vi "TFTLCD显示实验.vi"() -> ()   [LabVIEW 2011]
uses:
  <vilib>/STM32_DriverVI_Interface_F4/LCD/Brush Color_Index_F4.ctl
  <vilib>/STM32_DriverVI_Interface_F4/LCD/Font_Size_F4.ctl
  <vilib>/STM32_DriverVI_Interface_F4/LCD/Show_Mode_F4.ctl
  <vilib>/STM32_DriverVI_Interface_F4/LCD/Direction_F4.ctl
  <vilib>/STM32_DriverVI_Interface_F4/LCD/Backlight_F4.ctl
  <vilib>/STM32_DriverVI_Interface_F4/LCD/LCD_Init_F4.vi
panel:
  in  "Display Direction":T1
  in  "停止":bool
  in  "轨迹颜色":T2=enum."Red"
  in  "矩形填充颜色":T2=enum."Magenta（品红）"
  in  "Show_Mode":T3
  in  "Font_Size":T4=enum."Big_Font（16）"
  in  "字体颜色":T2=enum."Magenta（品红）"
  in  "清屏背景色":T2
  in  "String":string="dlw30@126.com"
  in  "Len":u16 max=320
  in  "U32 Number":u32=999999
  out "LCD_ID":u16 format="%x"
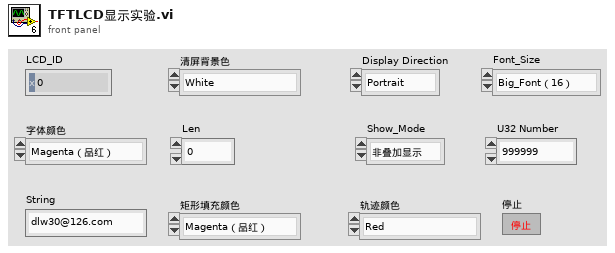
[diagram p1: front panel]
types:
  T1 = typedef "Direction_F4.ctl" = enum8{"Portrait", "Landscape"}
  T2 = typedef "Brush Color_Index_F4.ctl" = enum8{"White", "Black", "Blue", "Green_Blue", "Red", "Magenta（品红）", "Green", "Cyan（青色）", "Yellow", "Brown", "Brown_Red", "Gray", "Dark_Blue", "Light_Blue", "Gray_Blue", "Light_Green", "Light_Gray", "Light_Gray_Blue", "Light_Brown_Blue"}
  T3 = typedef "Show_Mode_F4.ctl" = enum8{"非叠加显示", "叠加显示"}
  T4 = typedef "Font_Size_F4.ctl" = enum8{"Small_Font（12）", "Big_Font（16）"}
  T5 = typedef "Backlight_F4.ctl" = enum8{"Light_Off", "Light_On"}
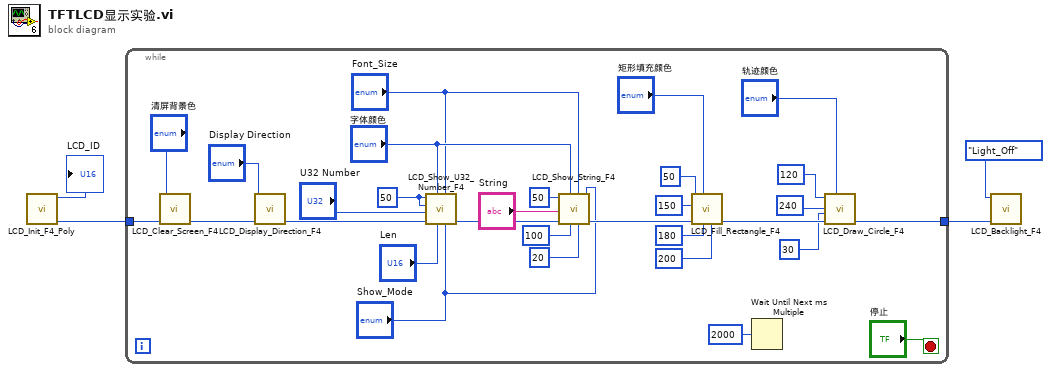
[diagram p0: block diagram]
diagram:
  n1 = call-poly <vilib>:"LCD_Init_F4_Poly.vi"() -> ("err_out"=w3:u8, "LCD_ID"=→"LCD_ID":u16)  [unwired: 10 in]
  n2 = while {
    tunnel: w3 -> [w34]
    tunnel: [w17] -> w2
    stop <- "停止" stop-if-true
    w31 = u16 50 ("X_Position")
    n3 = call <vilib>:"LCD_Clear_Screen_F4.vi"("err_in"=w34, "Brush Color"="清屏背景色") -> ("err_out"=w33:u8)  [unwired: 9 in]
    n4 = call <vilib>:"LCD_Display_Direction_F4.vi"("err_in"=w33, "Display Direction"="Display Direction") -> ("err_out"=w32:u8)  [unwired: 9 in]
    n5 = call <vilib>:"LCD_Show_U32_Number_F4.vi"("Show_Mode"="Show_Mode", "Font_Size"="Font_Size", "Len"="Len", "Brush Color"="字体颜色", "err_in"=w32, "U32 Number"="U32 Number", "Y_Position"=w31, "X_Position"=w31) -> ("err_out"=w28:u8)  [unwired: 3 in]
    n6 = call <vilib>:"LCD_Show_String_F4.vi"("Show_Mode"="Show_Mode", "Height"=u16 20, "Font_Size"="Font_Size", "Width"=u16 100, "Brush Color"="字体颜色", "err_in"=w28, "String"="String", "X_Position"=u16 50) -> ("err_out"=w25:u8)  [unwired: 3 in]
    n7 = call <vilib>:"LCD_Fill_Rectangle_F4.vi"("Y2_Position"=u16 200, "X2_Position"=u16 180, "Brush Color"="矩形填充颜色", "err_in"=w25, "Y1_Position"=u16 150, "X1_Position"=u16 50) -> ("err_out"=w18:u8)  [unwired: 5 in]
    n8 = Wait Until Next ms Multiple(millisecond multiple=u32 2000 ("毫秒倍数")) -> ()  [unwired: 1 out]
    n9 = call <vilib>:"LCD_Draw_Circle_F4.vi"("Brush Color"="轨迹颜色", "err_in"=w18, "R"=u16 30, "Y0_Position"=u16 240, "X0_Position"=u16 120) -> ("err_out"=w17:u8)  [unwired: 6 in]
  }
  n10 = call <vilib>:"LCD_Backlight_F4.vi"("err_in"=w2, "Backlight"=Backlight_F4."Light_Off") -> ()  [unwired: 9 in, 1 out]
